vi "Main-Main.vi"() -> ()   [LabVIEW 2016]
uses:
  <vilib>/myRIO/Instrument Drivers/Onboard IO/AI/typedefs/AI Reference.ctl
  <vilib>/myRIO/Common/Instrument Driver Framework/Utilities/typedefs/myRIO Generic Hardware Reference.ctl
  <vilib>/myRIO/Common/Instrument Driver Framework/Utilities/typedefs/Hardware Version Enum.ctl
  <vilib>/myRIO/Common/Instrument Driver Framework/Utilities/typedefs/myRIO v1.0 Reference.ctl
  <vilib>/myRIO/Common/Instrument Driver Framework/Utilities/typedefs/Generic FPGA Reference.ctl
  <vilib>/myRIO/Common/Instrument Driver Framework/myRIO v1.0/AI/typedefs/AI Channels List.ctl
  <vilib>/myRIO/Common/Instrument Driver Framework/myRIO v1.0/AI/typedefs/AI Channels Enum.ctl
  <vilib>/myRIO/Common/Instrument Driver Framework/Utilities/typedefs/Analog Scaling Constants List.ctl
  <vilib>/myRIO/Common/Instrument Driver Framework/Utilities/typedefs/Analog Scaling Constants.ctl
  <vilib>/userdefined/High Color/nirio_resource_hc.ctl
  <vilib>/myRIO/Common/Instrument Driver Framework/Utilities/vis/Is FPGA Ref Available.vi
  <vilib>/myRIO/Common/Instrument Driver Framework/myRIO v1.0/AI/vis/myRIO v1.1 Open AI.vi
  <vilib>/myRIO/Instrument Drivers/Onboard IO/AI/vis/Read.vi
  <vilib>/myRIO/Common/Instrument Driver Framework/Utilities/vis/Validate Channels.vi
  <vilib>/myRIO/Common/Instrument Driver Framework/myRIO v1.0/AI/vis/myRIO v1.0 Reserve AI.vi
  <vilib>/myRIO/Common/Instrument Driver Framework/myRIO v1.0/AI/vis/myRIO v1.0 Build MUX Configuration AI.vi
  <vilib>/myRIO/Common/Instrument Driver Framework/myRIO v1.0/Resource Manager/vis/myRIO v1.0 Reserve Channel List.vi
  <vilib>/myRIO/Common/Instrument Driver Framework/myRIO v1.0/Resource Manager/vis/myRIO v1.0 Reserve Channel.vi
  <vilib>/myRIO/Common/Instrument Driver Framework/myRIO v1.0/Resource Manager/vis/myRIO v1.0 Unreserve Channel.vi
  <vilib>/myRIO/Common/Instrument Driver Framework/myRIO v1.0/Resource Manager/vis/myRIO v1.0 Build Mutex Name.vi
  <vilib>/Utility/VariantDataType/GetNumericInfo.vi
  <vilib>/Utility/error.llb/Error Cluster From Error Code.vi
  <vilib>/myRIO/Common/Instrument Driver Framework/myRIO v1.0/myRIO v1.1 Open.vi
  <vilib>/myRIO/Common/Instrument Driver Framework/myRIO v1.0/AI/vis/myRIO v1.0 Get Scaling Constants AI.vi
  <vilib>/myRIO/Common/Instrument Driver Framework/Utilities/vis/IO Manager.vi
  <vilib>/myRIO/Common/Instrument Driver Framework/Utilities/vis/Configuration Manager.vi
  <vilib>/myRIO/Common/Instrument Driver Framework/myRIO v1.0/myRIO v1.0 Close.vi
  <vilib>/myRIO/Common/Instrument Driver Framework/myRIO v1.0/AI/vis/myRIO v1.0 Read AI.vi
  <vilib>/myRIO/Express VI/Onboard IO/AI/AI Express VI.xnode
  <vilib>/myRIO/Instrument Drivers/Onboard IO/AI/vis/myRIO AI Open.xnode
  <vilib>/myRIO/Instrument Drivers/Onboard IO/AI/AI.lvlib
panel:
  out "Ausgabe Strommessung":dbl
  in  "lowest":bool
  out "nicht beachten!":bool
  in  "IR or Linearray":bool
  in  "stop 2":bool
  in  "stop":bool
  out "Leistung":dbl
  out "Impulse pro Minute":dbl
  out "counter":dbl
  out "Drehzahl":dbl(knob) scale=0.0..15000.0
  out "Linefollow-array":bool[](array[boolean])
  out "Volt":dbl(knob) scale=6.0..8.4 scale format="%#_2g"
  out "Strom":dbl=-149.04557758721205 format="%#_4g"
  in  "Stop":bool
  in  "Geschwindigkeit":dbl(knob)=0.1402796355699434 scale=0.0..2.0
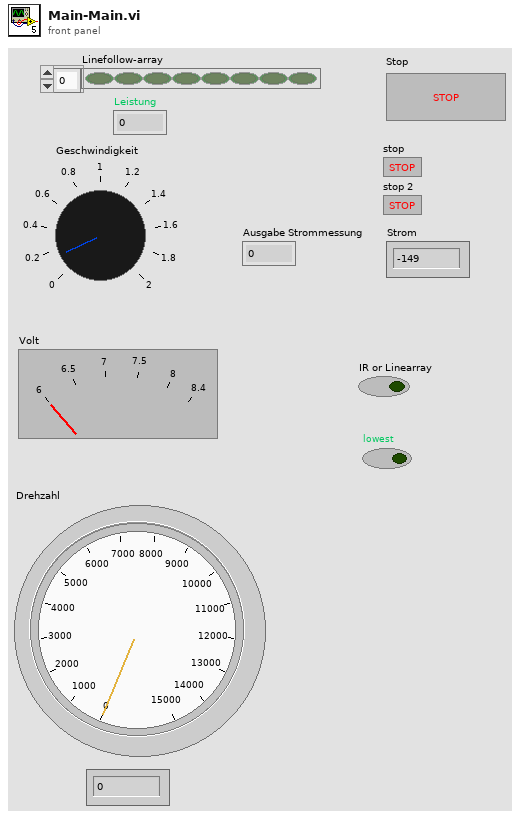
[diagram p1: front panel]
types:
  T1 = typedef "AI.lvlib/AI Reference.ctl" = cluster{"myRIO Reference":T2, "AI Channels List":T6, "AI Scaling Constants List":T8}
  T2 = typedef "myRIO Generic Hardware Reference.ctl" = cluster{"myRIO Model":T3, "myRIO Hardware Reference":T4}
  T3 = typedef "Hardware Version Enum.ctl" = enum16{"Unknown", "myRIO-1900", "myRIO-1950", "roboRIO", "NI ELVIS RIO CM"}
  T4 = typedef "myRIO v1.0 Reference.ctl" = cluster{"Generic FPGA Reference":T5, "Allow multiple opens":bool}
  T5 = typedef "Generic FPGA Reference.ctl" = refnum<k20>
  T6 = typedef "AI Channels List.ctl" = T7[]
  T7 = typedef "AI Channels Enum.ctl" = enum16{"Not Connected", "AudioIn/Left", "AudioIn/Right", "C/AI0", "C/AI1", "A/AI0", "A/AI1", "A/AI2", "A/AI3", "B/AI0", "B/AI1", "B/AI2", "B/AI3", "AI/AI0", "AI/AI1", "AI/AI2", "AI/AI3"}
  T8 = typedef "Analog Scaling Constants List.ctl" = T9[]
  T9 = typedef "Analog Scaling Constants.ctl" = cluster{"LSB Weight (Volts)":dbl, "Offset (Volts)":dbl, "Signed?":bool}
  T10 = typedef "nirio_resource_hc.ctl" = tag
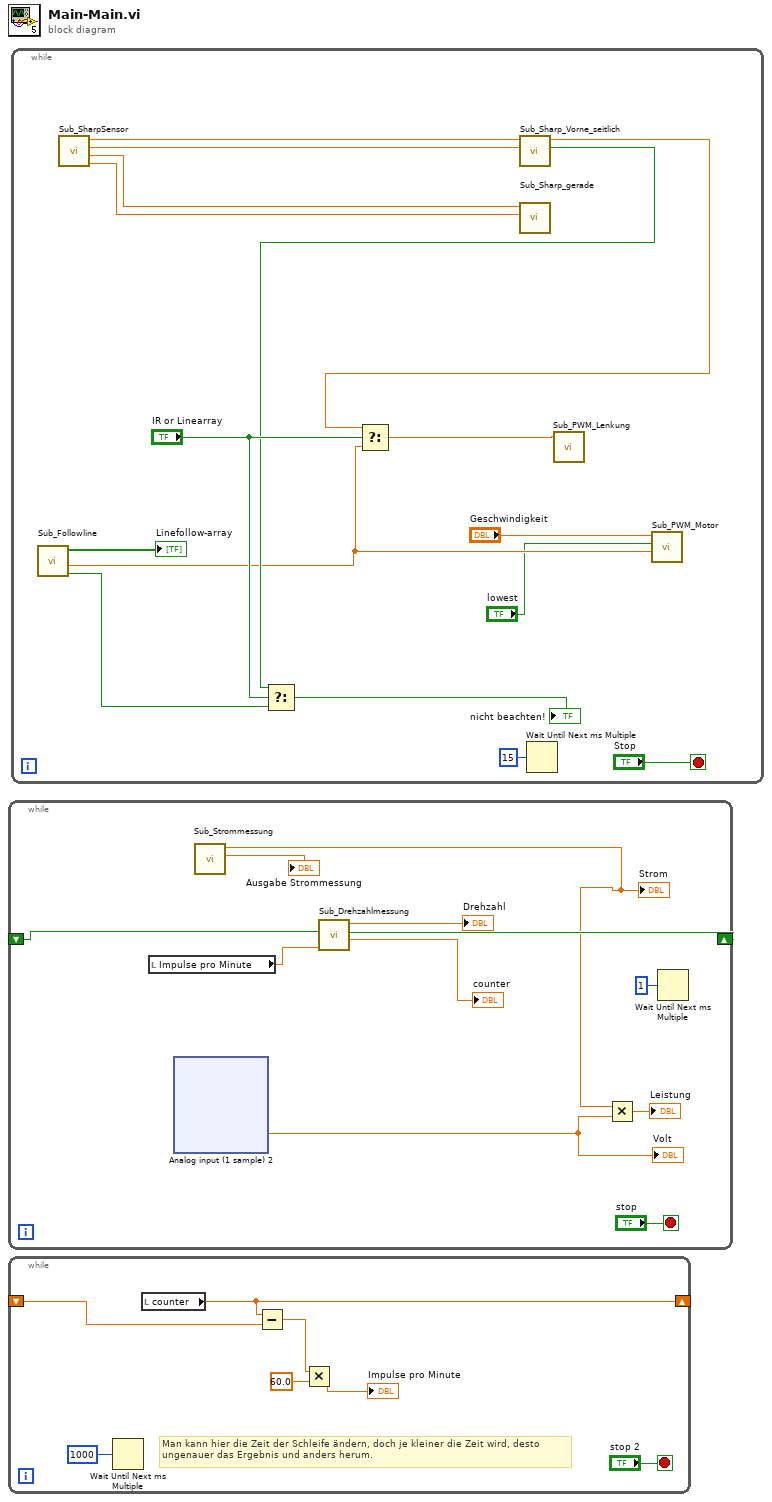
[diagram p0: block diagram]
diagram:
  n1 = while {
    shift-right: [w7] -> _
    shift-left: _ -> [w3]
    stop <- "stop" stop-if-true
    n2 = local read "Impulse pro Minute"() -> (w10:dbl)
    n3 = xnode "Analog input (1 sample) 2"() -> ("C/AI0 (AI0)"=w6:dbl)  [unwired: 1 in, 1 out]
    "Volt" <- w6
    n4 = call "Sub_Strommessung.vi"() -> ("Ausgabe Strommessung"=→"Ausgabe Strommessung":dbl, "Strom"=w2:dbl)  [unwired: 10 in]
    "Strom" <- w2
    n5 = call "Sub_Drehzahlmessung.vi"("Impuls per Minute"=w10, "in"=w3) -> ("counter"=→"counter":dbl, "out"=w7:bool, "Drehzahl"=→"Drehzahl":dbl)  [unwired: 6 in]
    n6 = Multiply(x=w2, y=w6) -> (x*y=→"Leistung":dbl)
    n7 = Wait Until Next ms Multiple(millisecond multiple=u32 1 ("milliseconds to wait")) -> ()  [unwired: 1 out]
  }
  n8 = while {
    shift-right: [w54] -> _
    shift-left: _ -> [w53]
    stop <- "stop 2" stop-if-true
    # "Man kann hier die Zeit der Schleife ändern, doch je kleiner die Zeit wird, desto\nungenauer das Ergebnis und anders herum."
    n9 = Wait Until Next ms Multiple(millisecond multiple=u32 1000 ("Vielfache von ms")) -> ()  [unwired: 1 out]
    n10 = local read "counter"() -> (w54:dbl)
    n11 = Subtract(x=w54, y=w53) -> (x-y=w50:dbl)
    n12 = Multiply(x=w50, y=60.0) -> (x*y=→"Impulse pro Minute":dbl)
  }
  n13 = while {
    stop <- "Stop" stop-if-true
    n14 = call "Sub_Followline.vi"() -> ("0 or 8?"=w66:bool, "Abweichung\nMittellinie"=w57:dbl, "Linefollow_Array"=→"Linefollow-array":bool[])  [unwired: 9 in]
    n15 = call "Sub_SharpSensor.vi"() -> ("links vorne"=w62:dbl, "rechts vorne"=w60:dbl, "gerade links"=w59:dbl, "gerade rechts"=w58:dbl)  [unwired: 3 in, 4 out]
    n16 = call "Sub_Sharp_Vorne_seitlich.vi"("rechts vorne"=w60, "links vorne"=w62) -> ("lower than 5?"=w63:bool, "Abweichung"=w61:dbl)  [unwired: 8 in]
    n17 = Select(t=w63, s="IR or Linearray", f=w66) -> (s? t:f=→"nicht beachten!":bool)
    n18 = Select(t=w61, s="IR or Linearray", f=w57) -> (s? t:f=w67:dbl)
    n19 = call "Sub_Sharp_gerade.vi"("gerade rechts"=w58, "gerade links"=w59) -> ()  [unwired: 9 in, 1 out]
    n20 = Wait Until Next ms Multiple(millisecond multiple=u32 15) -> ()  [unwired: 1 out]
    n21 = call "Sub_PWM_Lenkung.vi"("Abweichung/ process variable"=w67) -> ()  [unwired: 11 in]
    n22 = call "Sub_PWM_Motor.vi"("Abweichung"=w57, "lowest"="lowest", "Geschwindigkeit"="Geschwindigkeit") -> ()  [unwired: 9 in]
  }
